vi "Check for valid imei.vi"(8 "error in (no error)":errorcluster, 9 "Be verbose?":bool, 10 "Got Imei?":bool=TRUE, 11 "14 or 15 digit IMEI":string) -> (0 "error out":errorcluster, 1 "15 digit imei":string, 3 "Valid IMEI":bool)   [LabVIEW 2013]
doc: "Pass a 14 digit imei if you want a checkdigit calc'd and 15 digit imei returned.\nPass a 15 digit imei if you want the check digit checked. Valid imei will indicate if ok\nEnable verbose for error message pop ups"
panel:
  out "sum":i32
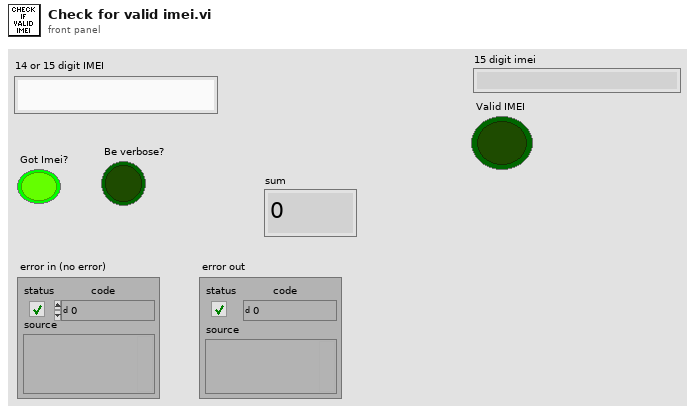
[diagram p1: front panel]
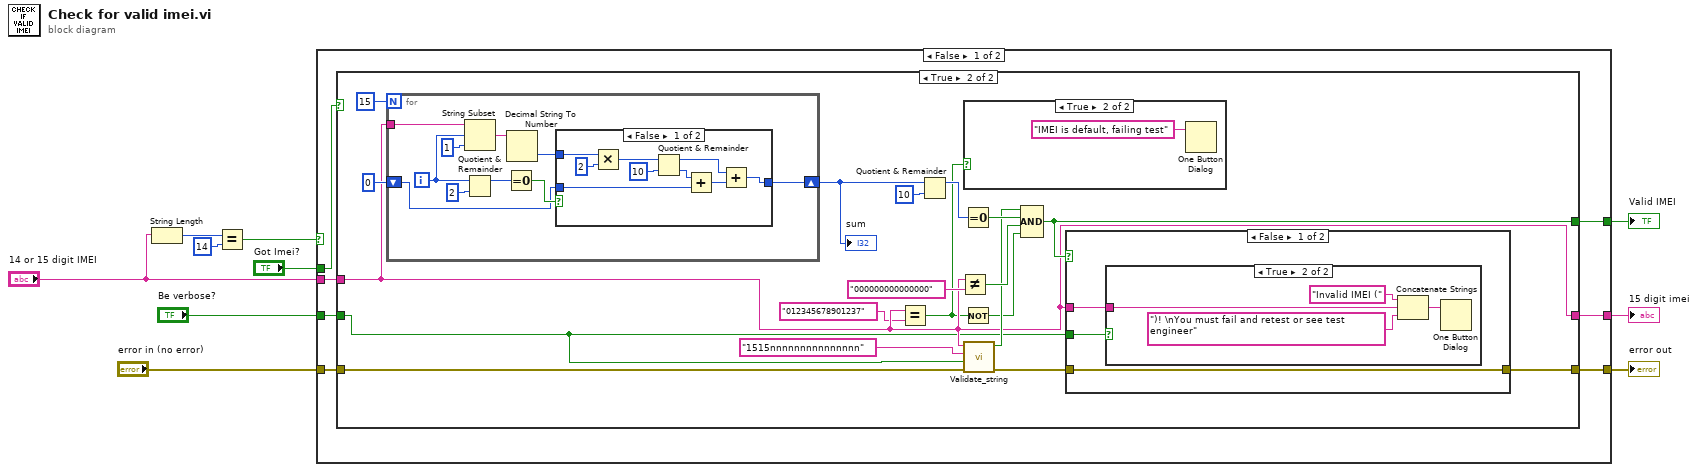
[diagram p0: block diagram]
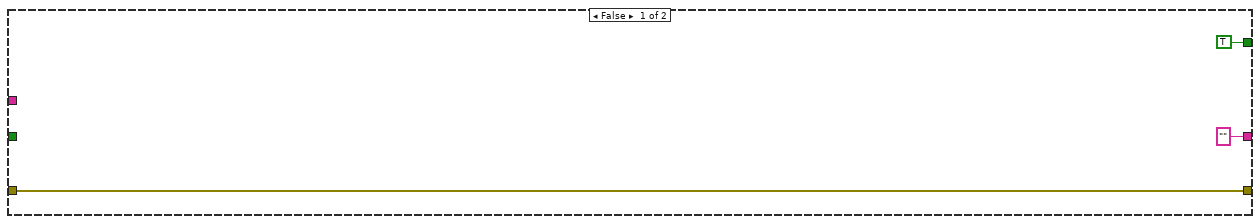
[diagram p2: hidden frame]
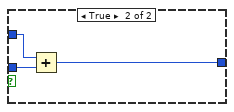
[diagram p6: hidden frame]
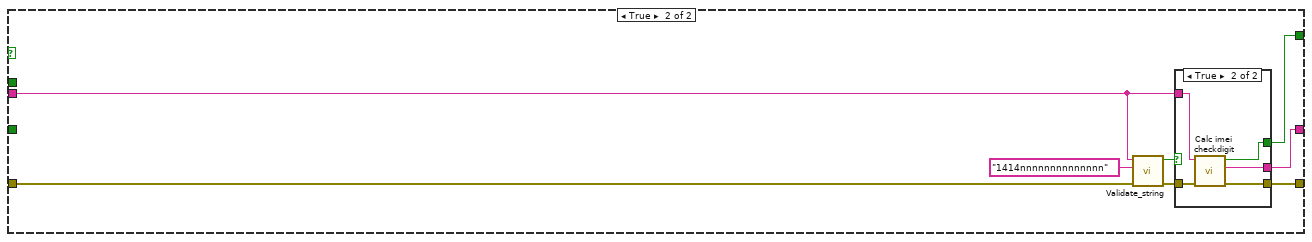
[diagram p7: hidden frame]
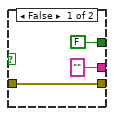
[diagram p8: hidden frame]
diagram:
  n1 = String Length(string="14 or 15 digit IMEI") -> (length=w4:i32)
  n2 = Equal?(x=w4, y=14) -> (x = y?=w2:bool)
  n3 = case shown="False" w2 {
    tunnel: [w17 w76] -> w10
    tunnel: "error in (no error)" -> [w16 w74]
    tunnel: "Got Imei?" -> [w15 _]
    tunnel: [w14 w78] -> w7
    tunnel: "Be verbose?" -> [w13 _]
    tunnel: "14 or 15 digit IMEI" -> [w12 w71]
    tunnel: [w11 w77] -> w1
    frame False {
      n4 = case shown="True" w15 {
        tunnel: [w19 w31] -> w17
        tunnel: w16 -> [w19 w29]
        tunnel: [TRUE w26] -> w14
        tunnel: w13 -> [_ w21]
        tunnel: w12 -> [_ w25]
        tunnel: ["" ("14 or 15 digit IMEI") w25] -> w11
        frame False {
        }
        frame True {
          n5 = for {
            N: 15 -> [_]
            tunnel: w25 -> [w58]
            shift-right: [w49] -> w37
            shift-left: 0 -> [w50]
            i -> [w56]
            n6 = String Subset(string=w58, offset (0)=w56, length (rest)=1 ("length (rest)")) -> (substring=w52:string)
            n7 = Quotient & Remainder(x=w56, y=2) -> (x-y*floor(x/y)=w54:i32)  [unwired: 1 out]
            n8 = Equal To 0?(x=w54) -> (x = 0?=w53:bool)
            n9 = Decimal String To Number(string=w52) -> (number=w51:i32)  [unwired: 2 in, 1 out]
            n10 = case shown="False" w53 {
              tunnel: w51 -> [w67 w70]
              tunnel: w50 -> [w62 w69]
              tunnel: [w59 w68] -> w49
              frame False {
                n11 = Multiply(x=w67, y=2) -> (x*y=w65:i32)
                n12 = Quotient & Remainder(x=w65, y=10) -> (x-y*floor(x/y)=w61:i32, floor(x/y)=w63:i32)
                n13 = Add(x=w63, y=w62) -> (x+y=w60:i32)
                n14 = Add(x=w61, y=w60) -> (x+y=w59:i32)
              }
              frame True {
                n15 = Add(x=w70, y=w69) -> (x+y=w68:i32)
              }
            }
          }
          "sum" <- w37
          n16 = Equal?(x=w25, y="012345678901237") -> (x = y?=w23:bool)
          n17 = Quotient & Remainder(x=w37, y=10) -> (x-y*floor(x/y)=w35:i32)  [unwired: 1 out]
          n18 = Not Equal?(x=w25, y="000000000000000") -> (x != y?=w33:bool)
          n19 = Equal To 0?(x=w35) -> (x = 0?=w32:bool)
          n20 = Not(x=w23) -> (.not. x?=w22:bool)
          n21 = case shown="True" w23 {
            frame False {
            }
            frame True {
              n22 = One Button Dialog(message="IMEI is default, failing test") -> ()  [unwired: 1 in, 1 out]
            }
          }
          n23 = call "Validate_string.vi"("error in (no error)"=w29, "Be verbose (F)"=w21, "String data format"="1515nnnnnnnnnnnnnnn", "String"=w25) -> ("error out"=w28:errorcluster, "String Valid"=w27:bool)  [unwired: 6 in]
          n24 = Compound Arithmetic op=AND(w27, w32, w33, w22) -> (w26:bool)
          n25 = case shown="False" w26 {
            tunnel: [w43 w48] -> w31
            tunnel: w28 -> [w43 w48]
            tunnel: w25 -> [w42 _]
            tunnel: w21 -> [w41 _]
            frame False {
              n26 = case shown="True" w41 {
                tunnel: w42 -> [_ w46]
                frame False {
                }
                frame True {
                  n27 = Concatenate Strings("Invalid IMEI (" ("message"), w46, ")! \nYou must fail and retest or see test engineer" ("message")) -> (w44:string)
                  n28 = One Button Dialog(message=w44) -> ()  [unwired: 1 in, 1 out]
                }
              }
            }
            frame True {
            }
          }
        }
      }
    }
    frame True {
      n29 = call "Validate_string.vi"("error in (no error)"=w74, "String data format"="1414nnnnnnnnnnnnnn", "String"=w71) -> ("error out"=w73:errorcluster, "String Valid"=w72:bool)  [unwired: 7 in]
      n30 = case shown="True" w72 {
        tunnel: w71 -> [_ w86]
        tunnel: [FALSE ("15 digit imei ok?") w85] -> w78
        tunnel: ["" ("15 digit imei") w84] -> w77
        tunnel: [w80 w83] -> w76
        tunnel: w73 -> [w80 w82]
        frame False {
        }
        frame True {
          n31 = call "Calc imei checkdigit.vi"("error in (no error)"=w82, "14 digit IMEI"=w86) -> ("error out"=w83:errorcluster, "15 digit imei"=w84:string, "15 digit imei ok?"=w85:bool)  [unwired: 7 in]
        }
      }
    }
  }
  "error out" <- w10
  "Valid IMEI" <- w7
  "15 digit imei" <- w1
